vi "16-ParseLiteralNibble.vi"(11 "BITS in in":bool[](array[boolean])) -> (1 "Last Nibble?":bool, 2 "Nibble":bool[](array[boolean]), 3 "BITS out":bool[](array[boolean]))   [LabVIEW 2019, in "16.lvlib"]
uses:
  16.lvlib
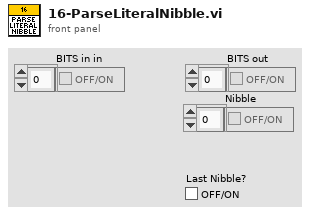
[diagram p1: front panel]
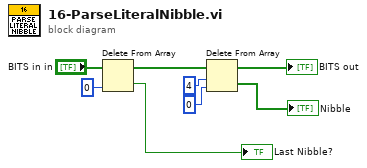
[diagram p0: block diagram]
diagram:
  n1 = Delete From Array(array="BITS in in", index=0) -> (deleted portion=→"Last Nibble?":bool, array with subset deleted=w5:bool[])  [unwired: 1 in]
  n2 = Delete From Array(array=w5, length=4, index=0) -> (deleted portion=→"Nibble":bool[], array with subset deleted=→"BITS out":bool[])
